vi "AlliGator Define Phasor References.vi"(0 "Phasor Graph":refnum<vi>, 1 "State Indicators Refnum":refnum<vi>, 5 "Phasor 1":T1, 7 "Phasor 2":T1, 9 "Phasor Frequency":dbl[unit], 11 "Error In":errorcluster) -> (4 "Reference Lifetime 1":dbl[unit], 6 "Reference Lifetime 2":dbl[unit], 8 "Phasor Reference 1":T1, 10 "Phasor Reference 2":T1, 15 "Error Out":errorcluster)   [LabVIEW 2021, in "AlliGator Phasor Ratio.lvlib"]
doc: "Reorders phasor references according to user preferences. Updates annotations in Phasor Graph."
uses:
  AlliGator Phasor Ratio.lvlib
  AlliGator State Indicator.ctl
  Phasor/Phasor (g, s).ctl
  AlliGator GUI.lvlib
  Phasor/Phasor.lvlib
panel:
  # "see the AlliGator License on the block diagram (Ctrl+E or Window:Show Block Diagram)"
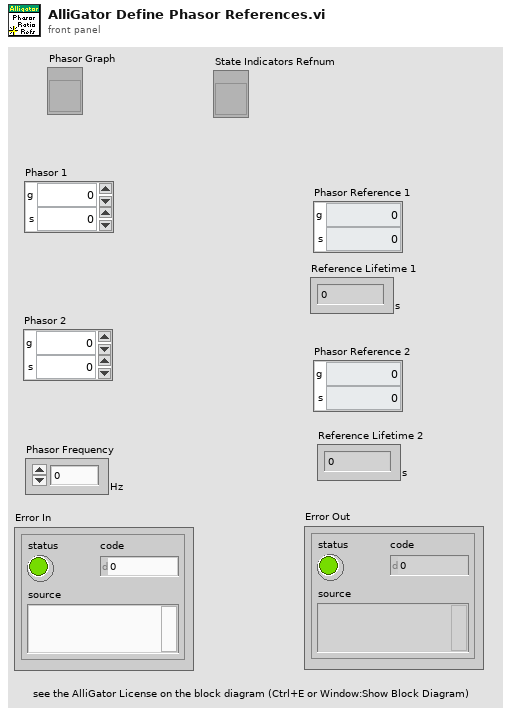
[diagram p1: front panel]
types:
  T1 = typedef "Phasor.lvlib/Phasor (g, s).ctl" = cluster{"g":dbl, "s":dbl}
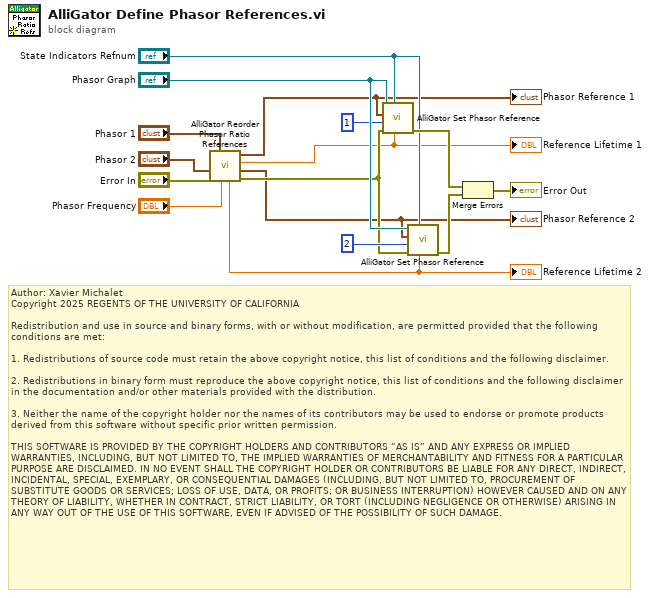
[diagram p0: block diagram]
diagram:
  # "Author: Xavier Michalet\nCopyright 2025 REGENTS OF THE UNIVERSITY OF CALIFORNIA\n\nRedistribution and use in source and binary forms, with or without modification, are permitted provided that the following conditions are met:\n\n1. Redistributions of source code must retain the above copyright notice, this list of conditions and the following disclaimer.\n\n2. Redistributions in binary form must reproduce the above copyright notice, this list of conditions and the following disclaimer in the documentation and/or other materials provided with the distribution.\n\n3. Neither the name of the copyright holder nor the names of its contributors may be used to endorse or promote products derived from this software without specific prior written permission.\n\nTHIS SOFTWARE IS PROVIDED BY THE COPYRIGHT HOLDERS AND CONTRIBUTORS “AS IS” AND ANY EXPRESS OR IMPLIED WARRANTIES, INCLUDING, BUT NOT LIMITED TO, THE IMPLIED WARRANTIES OF MERCHANTABILITY AND FITNESS FOR A PARTICULAR PURPOSE ARE DISCLAIMED. IN NO EVENT SHALL THE COPYRIGHT HOLDER OR CONTRIBUTORS BE LIABLE FOR ANY DIRECT, INDIRECT, INCIDENTAL, SPECIAL, EXEMPLARY, OR CONSEQUENTIAL DAMAGES (INCLUDING, BUT NOT LIMITED TO, PROCUREMENT OF SUBSTITUTE GOODS OR SERVICES; LOSS OF USE, DATA, OR PROFITS; OR BUSINESS INTERRUPTION) HOWEVER CAUSED AND ON ANY THEORY OF LIABILITY, WHETHER IN CONTRACT, STRICT LIABILITY, OR TORT (INCLUDING NEGLIGENCE OR OTHERWISE) ARISING IN ANY WAY OUT OF THE USE OF THIS SOFTWARE, EVEN IF ADVISED OF THE POSSIBILITY OF SUCH DAMAGE."
  n1 = call "AlliGator Reorder Phasor Ratio References.vi"("Phasor Frequency"="Phasor Frequency", "error in (no error)"="Error In", "Phasor 2"="Phasor 2", "Phasor 1"="Phasor 1") -> ("error out"=w8:errorcluster, "Reference 2"=w4:T1, "Phase Lifetime 1"=w2:dbl[unit], "Reference 1"=w5:T1, "Phase Lifetime 2"=w1:dbl[unit])  [unwired: 3 in]
  "Reference Lifetime 2" <- w1
  "Reference Lifetime 1" <- w2
  "Phasor Reference 1" <- w5
  "Phasor Reference 2" <- w4
  n2 = call "AlliGator Set Phasor Reference.vi"("Lifetime"=w2, "State Indicators Refnum"="State Indicators Refnum", "error in (no error)"=w8, "Reference Number"=1, "Plot Data Point"=w5, "Phasor Graph Refnum"="Phasor Graph") -> ("Error Out"=w11:errorcluster)  [unwired: 5 in]
  n3 = call "AlliGator Set Phasor Reference.vi"("Lifetime"=w1, "State Indicators Refnum"="State Indicators Refnum", "error in (no error)"=w8, "Reference Number"=2, "Plot Data Point"=w4, "Phasor Graph Refnum"="Phasor Graph") -> ("Error Out"=w15:errorcluster)  [unwired: 5 in]
  n4 = Merge Errors(w11, w15) -> (→"Error Out":errorcluster)
